vi "LakeShore Ramp.vi"(4 "Loop":bool, 6 "Parameter":bool=TRUE, 7 "Mapping":bool=TRUE, 8 "Time (Hr:Min:Sec)":dbl=540.0 format="%<%H:%M:%S>t", 9 "End Temp/Power":dbl=0.02 format="%.3p", 10 "Start Temp/Power":dbl=15.0 format="%.3p", 11 "VISA resource name":refnum<visa-resource-name>) -> ()   [LabVIEW 2020]
doc: "This VI will ramp the setpoint of the LakeShore Model 370 Temperature Controller logarithmically over the temperature range specified. Enter the values and run the VI. It will update the current temperature and the last value sent to the setpoint.\nScott Hannahs, <sth@magnet.fsu.edu> NHMFL-FSU, May 2003"
panel:
  out "dup VISA session":refnum<visa-resource-name>
  out "Last Value Sent":dbl=15.0 format="%.3p"
  out "Current\nTemp/Power":dbl=15.0 format="%.3p"
  in  "stop":bool
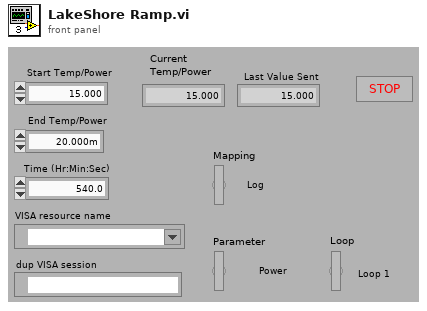
[diagram p1: front panel]
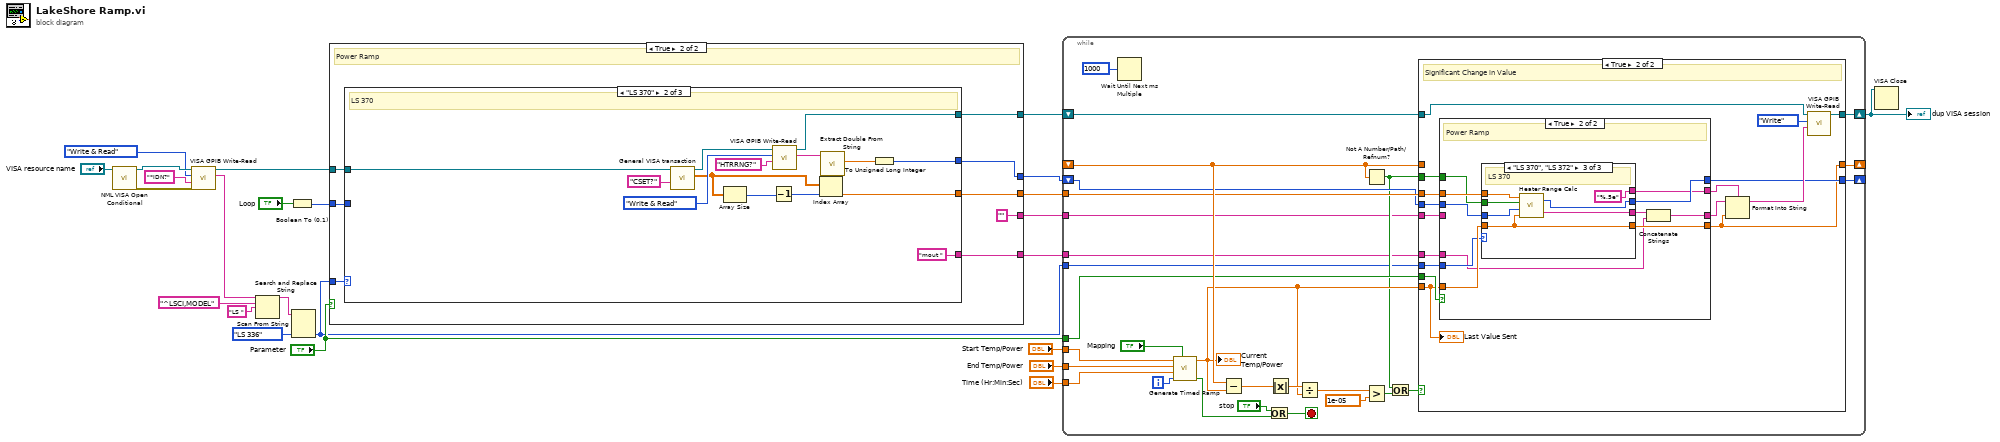
[diagram p0: block diagram]
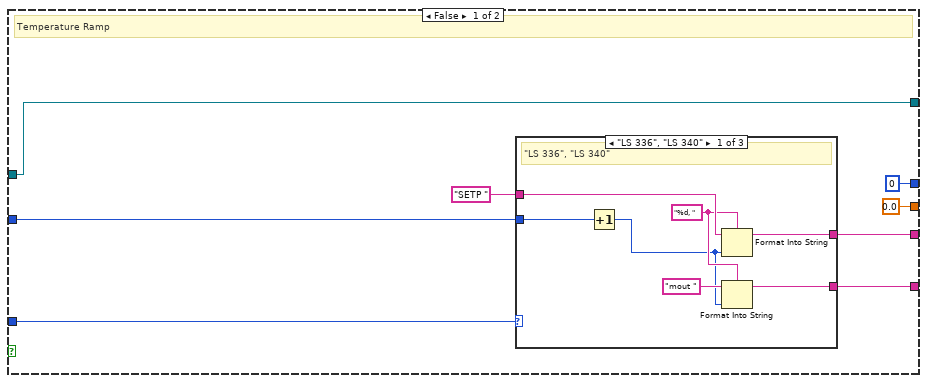
[diagram p2: hidden frame]
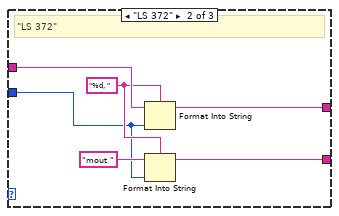
[diagram p3: hidden frame]
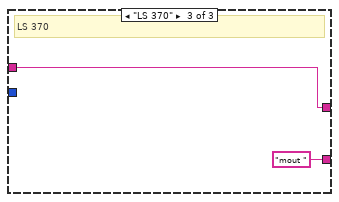
[diagram p4: hidden frame]
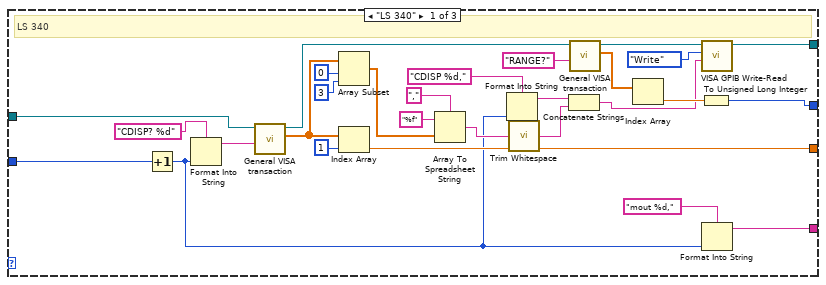
[diagram p5: hidden frame]
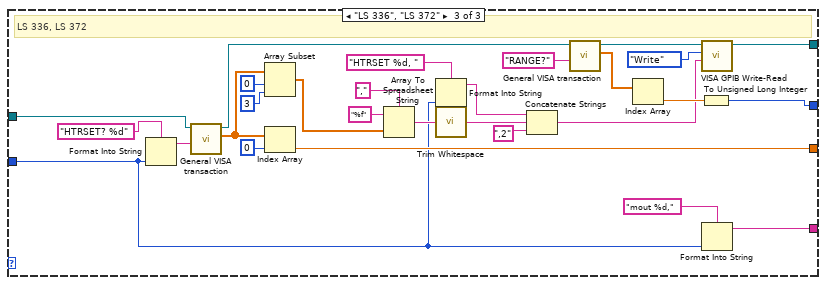
[diagram p6: hidden frame]
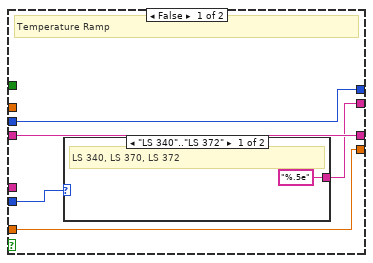
[diagram p8: hidden frame]
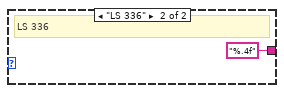
[diagram p9: hidden frame]
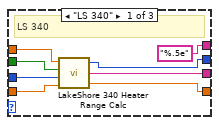
[diagram p10: hidden frame]
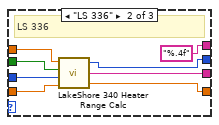
[diagram p11: hidden frame]
diagram:
  n1 = call "NML VISA Open Conditional.vi"("VISA resource name"="VISA resource name") -> ("error out"=w9:errorcluster, "dup VISA Session"=w10:refnum<visa-resource-name>)  [unwired: 8 in, 1 out]
  n2 = call "VISA GPIB Write-Read.vi"("error in (no error)"=w9, "Command"="*IDN?", "Action"=enum16{"Write", "Read", "Write & Read"}."Write & Read", "VISA resource name"=w10) -> ("String Returned"=w3:string, "dup VISA Session"=w11:refnum<visa-resource-name>)  [unwired: 4 in, 2 out]
  n3 = Search and Replace String(input string=w3, search string="^LSCI,MODEL", replace string="LS " ("replace string (\"\")")) -> (result string=w6:string)  [unwired: 5 in, 3 out]
  n4 = Boolean To (0,1)(Boolean="Loop") -> (0, 1=w12:i16)
  n5 = Scan From String(input string=w6, default 1=enum16{"LS 336", "LS 340", "LS 370", "LS 372"}."LS 336" ("Controller Model 2")) -> (output 1=w1:enum16{"LS 336", "LS 340", "LS 370", "LS 372"})  [unwired: 3 in, 3 out]
  n6 = case shown="True" "Parameter" {
    tunnel: w1 -> [w32 w55]
    tunnel: [w31 "" ("format string")] -> w21
    tunnel: w12 -> [w30 w49]
    tunnel: w11 -> [w28 w54]
    tunnel: [u32 0 w52] -> w19
    tunnel: [w28 w53] -> w18
    tunnel: [0.0 w51] -> w17
    tunnel: [w25 w48] -> w13
    frame False {
      # "Temperature Ramp"
      n7 = case shown="\"LS 336\", \"LS 340\"" w32 {
        tunnel: [w39 w45 w47] -> w31
        tunnel: w30 -> [w35 w40 _]
        tunnel: "SETP " ("format string") -> [w38 w44 w47]
        tunnel: [w36 w42 "mout " ("string")] -> w25
        frame "LS 336", "LS 340" {
          w34 = "%d, " ("format string")
          # "\"LS 336\", \"LS 340\""
          n8 = Increment(x=w35) -> (x+1=w33:i16)
          n9 = Format Into String(format string=w34, initial string=w38, w33) -> (resulting string=w39:string)  [unwired: 1 in, 1 out]
          n10 = Format Into String(format string=w34, initial string="mout " ("string"), w33) -> (resulting string=w36:string)  [unwired: 1 in, 1 out]
        }
        frame "LS 372" {
          w41 = "%d, " ("format string")
          # "\"LS 372\""
          n11 = Format Into String(format string=w41, initial string=w44, w40) -> (resulting string=w45:string)  [unwired: 1 in, 1 out]
          n12 = Format Into String(format string=w41, initial string="mout " ("string"), w40) -> (resulting string=w42:string)  [unwired: 1 in, 1 out]
        }
        frame "LS 370" {
          # "LS 370"
        }
      }
    }
    frame True {
      # "Power Ramp"
      n13 = case shown="\"LS 370\"" w55 {
        tunnel: w54 -> [w68 w88 w110]
        tunnel: [w65 w86 w107] -> w53
        tunnel: [w67 w87 w109] -> w52
        tunnel: [w66 w85 w108] -> w51
        tunnel: w49 -> [w60 _ w100]
        tunnel: [w61 "mout " w102] -> w48
        frame "LS 340" {
          # "LS 340"
          n14 = Increment(x=w60) -> (x+1=w58:i16)
          n15 = Format Into String(format string="CDISP? %d" ("Command String"), w58) -> (resulting string=w57:string)  [unwired: 2 in, 1 out]
          n16 = call "General VISA transaction.vi"("Command String"=w57, "VISA Session"=w68) -> ("Measurement"=w82:dbl[], "dup VISA Session"=w75:refnum<visa-resource-name>)  [unwired: 4 in, 4 out]
          n17 = Array Subset(array=w82, index=0, length=3 ("new element/subarray")) -> (w78:dbl[])
          n18 = Index Array(array=w82, index=1) -> (element=w66:dbl)
          n19 = Array To Spreadsheet String(delimiter (Tab)=",", array=w78, 3:"%f" ("format string")) -> (spreadsheet string=w79:string)
          n20 = Format Into String(format string="CDISP %d," ("Command String"), w58) -> (resulting string=w56:string)  [unwired: 2 in, 1 out]
          n21 = call <vilib>:"Trim Whitespace.vi"("string"=w79) -> ("trimmed string"=w63:string)  [unwired: 1 in]
          n22 = Concatenate Strings(w56, w63) -> (w69:string)
          n23 = call "General VISA transaction.vi"("Command String"="RANGE?" ("String to Write"), "VISA Session"=w75) -> ("Measurement"=w73:dbl[], "dup VISA Session"=w71:refnum<visa-resource-name>)  [unwired: 4 in, 4 out]
          n24 = Index Array(array=w73) -> (element=w72:dbl)  [unwired: 1 in]
          n25 = To Unsigned Long Integer(number=w72) -> (unsigned 32bit integer=w67:u32)
          n26 = call "VISA GPIB Write-Read.vi"("Command"=w69, "Action"=enum16{"Write", "Read", "Write & Read"}."Write", "VISA resource name"=w71) -> ("dup VISA Session"=w65:refnum<visa-resource-name>)  [unwired: 5 in, 3 out]
          n27 = Format Into String(format string="mout %d," ("string"), w58) -> (resulting string=w61:string)  [unwired: 2 in, 1 out]
        }
        frame "LS 370" {
          # "LS 370"
          n28 = call "General VISA transaction.vi"("Command String"="CSET?", "VISA Session"=w88) -> ("Measurement"=w91:dbl[], "dup VISA Session"=w94:refnum<visa-resource-name>)  [unwired: 4 in, 4 out]
          n29 = Array Size(array=w91) -> (size(s)=w92:i32)
          n30 = Decrement(x=w92) -> (x-1=w90:i32)
          n31 = call "VISA GPIB Write-Read.vi"("Command"="HTRRNG?" ("String to Write"), "Action"=enum16{"Write", "Read", "Write & Read"}."Write & Read", "VISA resource name"=w94) -> ("String Returned"=w93:string, "dup VISA Session"=w86:refnum<visa-resource-name>)  [unwired: 5 in, 2 out]
          n32 = Index Array(array=w91, index=w90) -> (element=w85:dbl)
          n33 = call "Extract Double From String.vi"("string"=w93) -> ("floating pt. number"=w89:dbl)  [unwired: 3 in, 3 out]
          n34 = To Unsigned Long Integer(number=w89) -> (unsigned 32bit integer=w87:u32)
        }
        frame "LS 336", "LS 372" {
          # "LS 336, LS 372"
          n35 = Format Into String(format string="HTRSET? %d" ("Command String"), w100) -> (resulting string=w105:string)  [unwired: 2 in, 1 out]
          n36 = call "General VISA transaction.vi"("Command String"=w105, "VISA Session"=w110) -> ("Measurement"=w124:dbl[], "dup VISA Session"=w117:refnum<visa-resource-name>)  [unwired: 4 in, 4 out]
          n37 = Array Subset(array=w124, index=0, length=3 ("new element/subarray")) -> (w120:dbl[])
          n38 = Index Array(array=w124, index=0) -> (element=w108:dbl)
          n39 = Array To Spreadsheet String(delimiter (Tab)=",", array=w120, 3:"%f" ("format string")) -> (spreadsheet string=w121:string)
          n40 = Format Into String(format string="HTRSET %d, " ("Command String"), w100) -> (resulting string=w99:string)  [unwired: 2 in, 1 out]
          n41 = call <vilib>:"Trim Whitespace.vi"("string"=w121) -> ("trimmed string"=w104:string)  [unwired: 1 in]
          n42 = Concatenate Strings(w99, w104, ",2" ("string")) -> (w111:string)
          n43 = call "General VISA transaction.vi"("Command String"="RANGE?" ("String to Write"), "VISA Session"=w117) -> ("Measurement"=w115:dbl[], "dup VISA Session"=w113:refnum<visa-resource-name>)  [unwired: 4 in, 4 out]
          n44 = Index Array(array=w115) -> (element=w114:dbl)  [unwired: 1 in]
          n45 = To Unsigned Long Integer(number=w114) -> (unsigned 32bit integer=w109:u32)
          n46 = call "VISA GPIB Write-Read.vi"("Command"=w111, "Action"=enum16{"Write", "Read", "Write & Read"}."Write", "VISA resource name"=w113) -> ("dup VISA Session"=w107:refnum<visa-resource-name>)  [unwired: 5 in, 3 out]
          n47 = Format Into String(format string="mout %d," ("string"), w100) -> (resulting string=w102:string)  [unwired: 2 in, 1 out]
        }
      }
    }
  }
  n48 = while {
    shift-right: [w145] -> _
    shift-left: _ -> [w143]
    tunnel: "End Temp/Power" -> [w141]
    tunnel: "Start Temp/Power" -> [w142]
    tunnel: "Time (Hr:Min:Sec)" -> [w140]
    tunnel: w21 -> [w128]
    shift-right: [w130] -> _
    shift-left: w19 -> [w131]
    shift-right: [w134] -> w14
    shift-left: w18 -> [w135]
    tunnel: w17 -> [w132]
    tunnel: "Parameter" -> [w133]
    tunnel: w1 -> [w127]
    tunnel: w13 -> [w126]
    i -> [w138]
    stop <- w151 stop-if-true
    n49 = Wait Until Next ms Multiple(millisecond multiple=u32 1000) -> ()  [unwired: 1 out]
    n50 = call "Generate Timed Ramp.vi"("Log"="Mapping", "Point #"=w138, "Time (Hr:Min:Sec)"=w140, "Stop"=w141, "Start"=w142) -> ("Stop"=w136:bool, "Output"=w137:dbl)  [unwired: 2 out]
    "Current\nTemp/Power" <- w137
    n51 = Subtract(x=w143, y=w137) -> (x-y=w150:dbl)
    n52 = Or(x="stop", y=w136) -> (x .or. y?=w151:bool)
    n53 = Absolute Value(x=w150) -> (abs(x)=w149:dbl)
    n54 = Divide(x=w149, y=w137) -> (x/y=w148:dbl)
    n55 = Not A Number/Path/Refnum?(number/path/refnum=w143) -> (NaN/Path/Refnum?=w129:bool)
    n56 = Greater?(x=w148, y=1e-05) -> (0:w146:bool)
    n57 = Or(x=w129, y=w146) -> (x .or. y?=w144:bool)
    n58 = case shown="True" w144 {
      tunnel: w137 -> [_ w161]
      tunnel: [w156 w160] -> w145
      tunnel: w143 -> [w156 _]
      tunnel: w135 -> [w155 w170]
      tunnel: [w155 w169] -> w134
      tunnel: w133 -> [_ w168]
      tunnel: w132 -> [_ w166]
      tunnel: w131 -> [w154 w165]
      tunnel: [w154 w164] -> w130
      tunnel: w129 -> [_ w163]
      tunnel: w128 -> [_ w162]
      tunnel: w127 -> [_ w159]
      tunnel: w126 -> [_ w158]
      frame False {
        # "Value Not Changed"
      }
      frame True {
        # "Significant Change in Value"
        n59 = case shown="True" w168 {
          tunnel: [w176 w186] -> w167
          tunnel: w166 -> [_ w190]
          tunnel: w165 -> [w177 w188]
          tunnel: w161 -> [w175 w184]
          tunnel: [w177 w187] -> w164
          tunnel: w163 -> [_ w185]
          tunnel: w162 -> [w176 _]
          tunnel: [w175 w183] -> w160
          tunnel: w159 -> [w173 w182]
          tunnel: w158 -> [_ w181]
          tunnel: [w174 w180] -> w157
          frame False {
            # "Temperature Ramp"
            n60 = case shown="\"LS 340\"..\"LS 372\"" w173 {
              tunnel: ["%.5e" ("format string") "%.4f" ("format string")] -> w174
              frame "LS 340".."LS 372" {
                # "LS 340, LS 370, LS 372"
              }
              frame "LS 336" {
                # "LS 336"
              }
            }
          }
          frame True {
            # "Power Ramp"
            n61 = case shown="\"LS 370\", \"LS 372\"" w182 {
              tunnel: w190 -> [w195 w203 w213]
              tunnel: [w193 w201 w212] -> w189
              tunnel: w188 -> [w197 w205 w211]
              tunnel: [w194 w202 w210] -> w187
              tunnel: w185 -> [w196 w204 w209]
              tunnel: w184 -> [w198 w206 w208]
              tunnel: [w192 w200 w208] -> w183
              tunnel: ["%.5e" ("format string") "%.4f" ("format string") "%.5e" ("format string")] -> w180
              frame "LS 340" {
                # "LS 340"
                n62 = call "LakeShore 340 Heater Range Calc.vi"("Power"=w198, "Heater Range"=w197, "Start Control?"=w196, "Resistance"=w195) -> ("Percent Power Out"=w192:dbl, "Command"=w193:string, "Heater Range Out"=w194:u32)
              }
              frame "LS 336" {
                # "LS 336"
                n63 = call "LakeShore 340 Heater Range Calc.vi"("Power"=w206, "Heater Range"=w205, "Start Control?"=w204, "Resistance"=w203) -> ("Percent Power Out"=w200:dbl, "Command"=w201:string, "Heater Range Out"=w202:u32)
              }
              frame "LS 370", "LS 372" {
                # "LS 370"
                n64 = call "Heater Range Calc.vi"("Power"=w208, "Heater Range"=w211, "Start Control?"=w209, "Resistance"=w213) -> ("Command"=w212:string, "Heater Range Out"=w210:u32)
              }
            }
            n65 = Concatenate Strings(w189, w181) -> (w186:string)
          }
        }
        n66 = Format Into String(format string=w157, initial string=w167, w160) -> (resulting string=w171:string)  [unwired: 1 in, 1 out]
        n67 = call "VISA GPIB Write-Read.vi"("Command"=w171, "Action"=enum16{"Write", "Read", "Write & Read"}."Write", "VISA resource name"=w170) -> ("dup VISA Session"=w169:refnum<visa-resource-name>)  [unwired: 5 in, 3 out]
        "Last Value Sent" <- w161
      }
    }
  }
  "dup VISA session" <- w14
  n68 = VISA Close(VISA resource name=w14) -> ()  [unwired: 1 in, 1 out]
